vi "GEN_Read Picture File.vi"(8 "error in":errorcluster caption="错误输入（无错误）", 11 "file in":path) -> (0 "error out":errorcluster, 2 "pic out":picture caption="空图片")   [LabVIEW 2016]
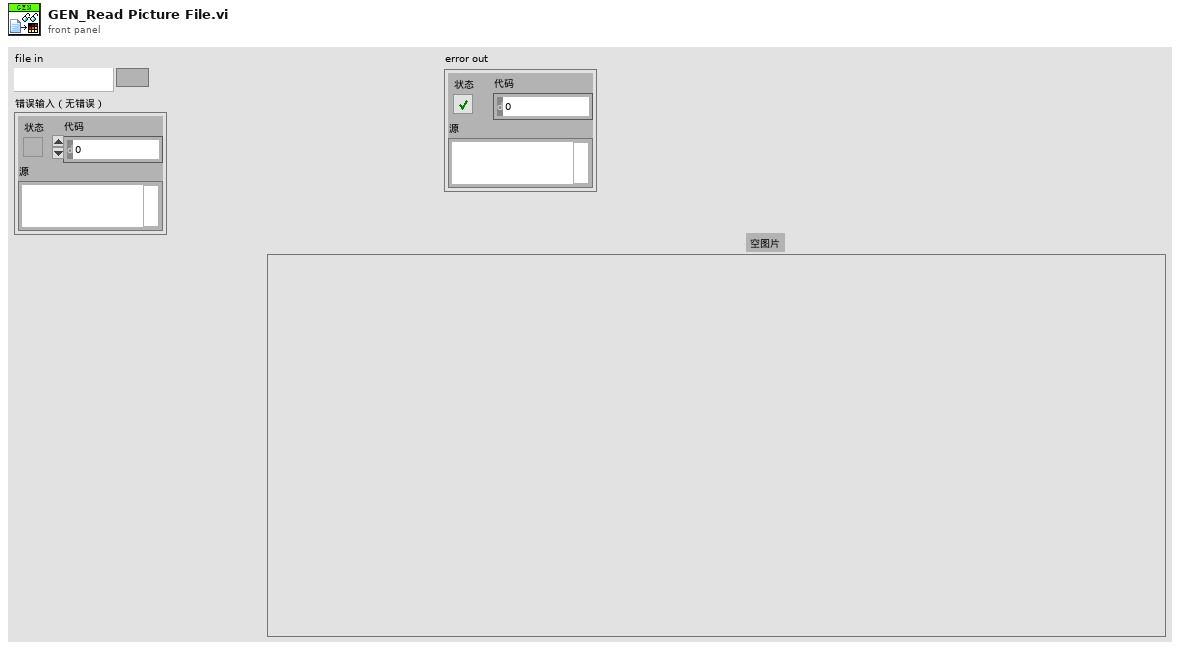
[diagram p1: front panel]
types:
  T1 = typedef "imagedata.ctl" = cluster{"image type":i32, "image depth":i32, "image":u8[], "mask":u8[], "colors":u32[], "Rectangle":cluster{"left":i16, "top":i16, "right":i16, "bottom":i16}}
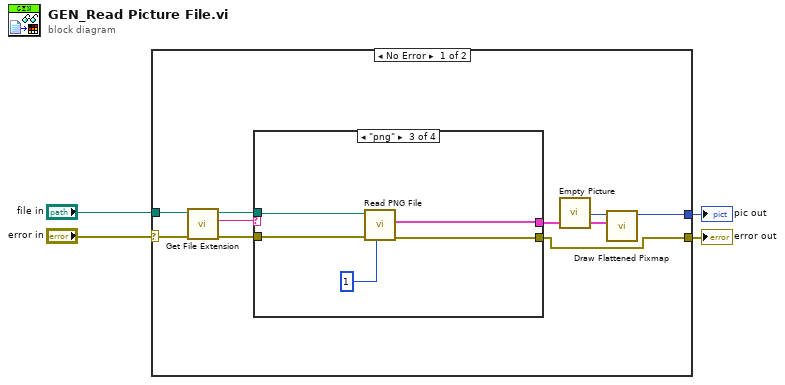
[diagram p0: block diagram]
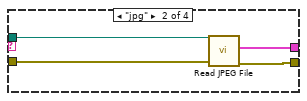
[diagram p3: hidden frame]
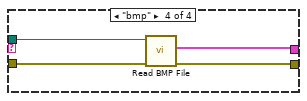
[diagram p4: hidden frame]
diagram:
  n1 = case shown="No Error" "error in" {
    selector: "error in" -> [w12 w28]
    tunnel: "file in" -> [w13 _]
    tunnel: [w6 _] -> w2
    tunnel: [w5 w28] -> w1
    frame No Error {
      n2 = call <vilib>:"Get File Extension.vi"("error in (no error)"=w12, "file"=w13) -> ("error out"=w10:errorcluster, "lowercase file extension"=w11:string, "dup file"=w9:path)  [unwired: 5 in, 2 out]
      n3 = case shown="\"png\"" w11 {
        tunnel: w10 -> [w14 w18 w23 w27]
        tunnel: w9 -> [_ w17 w20 w24]
        tunnel: [_ w16 w21 w25] -> w8
        tunnel: [w14 w15 w22 w26] -> w5
        frame Default {
        }
        frame "jpg" {
          n4 = call <vilib>:"Read JPEG File.vi"("error in (no error)"=w18, "path to JPEG file"=w17) -> ("error out"=w15:errorcluster, "image data"=w16:T1)  [unwired: 7 in, 1 out]
        }
        frame "png" {
          n5 = call <vilib>:"Read PNG File.vi"("Transparency Thresh"=u8 1, "error in (no error)"=w23, "path to PNG file"=w20) -> ("error out"=w22:errorcluster, "image data"=w21:T1)  [unwired: 6 in, 1 out]
        }
        frame "bmp" {
          n6 = call <vilib>:"Read BMP File.vi"("error in (no error)"=w27, "path to BMP file"=w24) -> ("error out"=w26:errorcluster, "image data"=w25:T1)  [unwired: 7 in, 1 out]
        }
      }
      n7 = call "Empty Picture"() -> ("empty picture"=w7:picture)
      n8 = call <vilib>:"Draw Flattened Pixmap.vi"("image data"=w8, "picture"=w7) -> ("new picture"=w6:picture)  [unwired: 7 in]
    }
    frame Error {
    }
  }
  "pic out" <- w2
  "error out" <- w1
